vi "_Get Target Object (Comm).vi"(8 "error in (no error)":errorcluster, 11 "Interface in":refnum<class "IUnknown.lvclass">) -> (0 "error out":errorcluster, 2 "Target Object":refnum<class "Interfaceable.lvclass">, 3 "Interface out":refnum<class "IUnknown.lvclass">)   [LabVIEW 2009, in "IUnknown.lvclass"]
doc: "Returns an object reference to the target object. This vi is called only by Interfaceable:GetInterface."
uses:
  IUnknown.lvclass
  Interfaceable Class/Interfaceable.lvclass
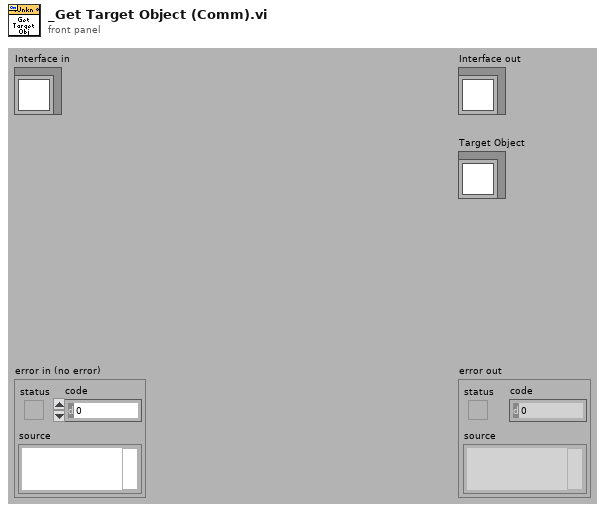
[diagram p1: front panel]
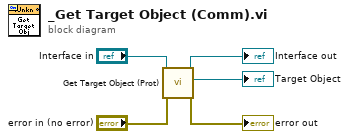
[diagram p0: block diagram]
diagram:
  n1 = call "Get Target Object (Prot).vi"("error in (no error)"="error in (no error)", "IUnknown in"="Interface in") -> ("error out"=→"error out":errorcluster, "Target Object"=→"Target Object":refnum<class "Interfaceable.lvclass">, "IUnknown out"=→"Interface out":refnum<class "IUnknown.lvclass">)  [unwired: 7 in]
